vi "Read-Role.vi"(11 "UDP_Config in":refnum<class "UDP_Config.lvclass">) -> (2 "Role":T1, 3 "UDP_Config out":refnum<class "UDP_Config.lvclass">)   [LabVIEW 2021, in "UDP_Config.lvclass"]
uses:
  UDP_Config.lvclass
  Control/Role.ctl
  UDP_Config.lvclass/UDP_Config.ctl
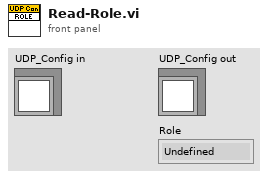
[diagram p1: front panel]
types:
  T1 = typedef "Role.ctl" = enum16{"Undefined", "Sender", "Receiver"}
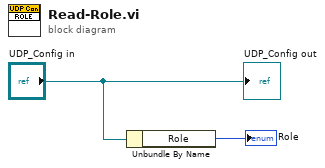
[diagram p0: block diagram]
diagram:
  n1 = Unbundle By Name("UDP_Config in") -> ("Role"=→"Role":T1)
  "UDP_Config out" <- "UDP_Config in"
